vi "Read Write Config File.vi"(4 "Operation":enum16{"Read", "Write"}(ring)=enum."Write", 6 "Config File":T1=enum."General", 8 "error in (no error)":errorcluster, 11 "Section-Key-Value In":string[][](array[string])) -> (0 "error out":errorcluster, 2 "Section-Key-Value Out":string[][](array[string]))   [LabVIEW 2020]
uses:
  Control/Config File Selection.ctl
  <vilib>/Utility/config.llb/Read Key (String).vi
  <vilib>/Utility/config.llb/Write Key (String).vi
  <vilib>/Utility/config.llb/NI_LVConfig.lvlib
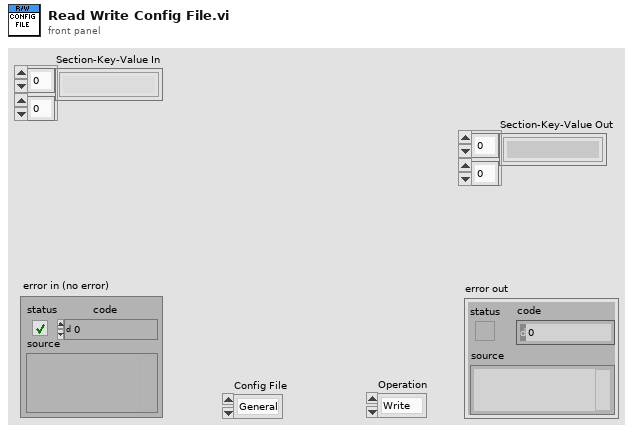
[diagram p1: front panel]
types:
  T1 = typedef "Config File Selection.ctl" = enum16{"Modbus", "SQL", "General"}
  T2 = enum32{"invalid app kind", "Development System", "Run Time System", "Student Edition", "Embedded LabVIEW", "Evaluation", "Custom"}
  T3 = typedef "NI_LVConfig.lvlib/Config Data RefNum.ctl" = refnum<k1>
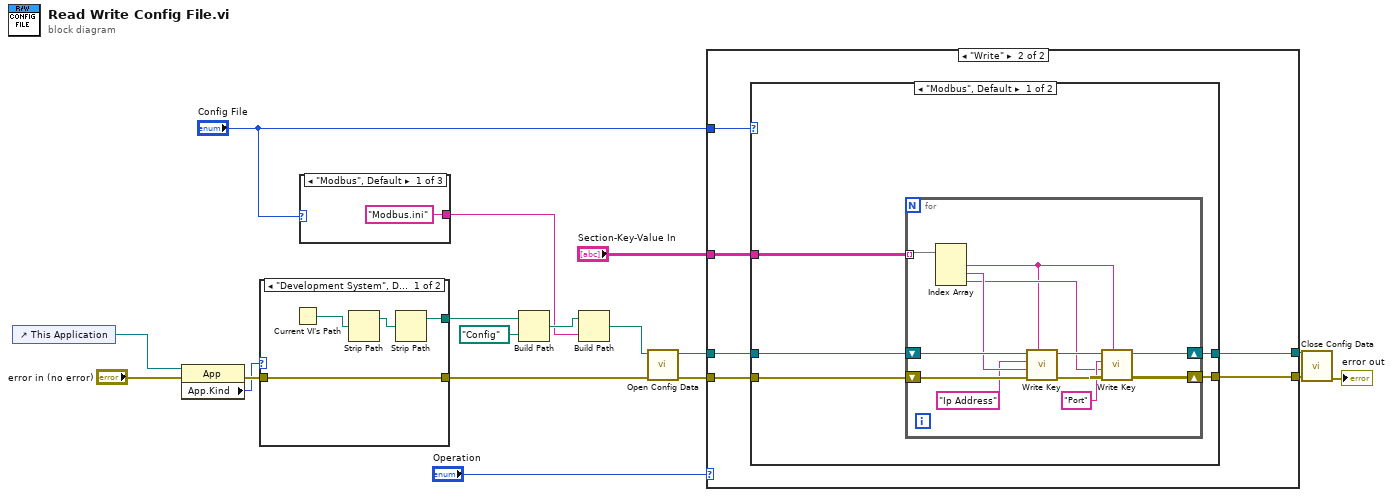
[diagram p0: block diagram]
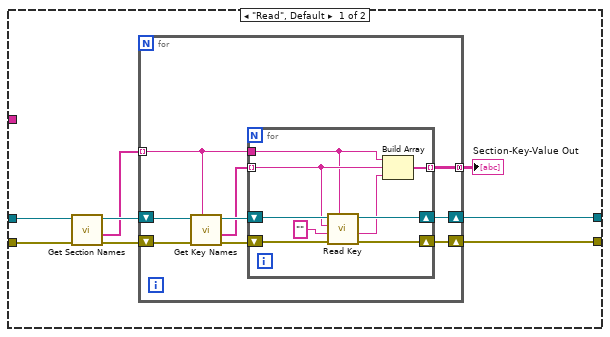
[diagram p2: hidden frame]
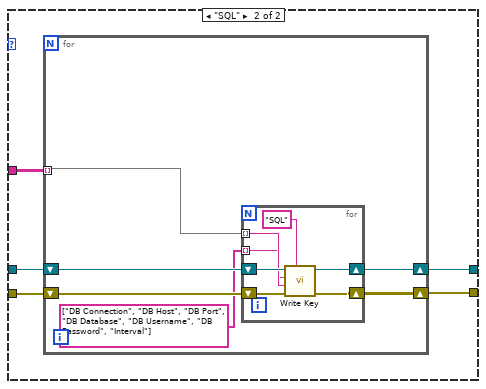
[diagram p3: hidden frame]
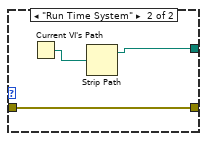
[diagram p4: hidden frame]
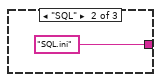
[diagram p5: hidden frame]
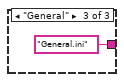
[diagram p6: hidden frame]
diagram:
  n1 = control-ref of="This Application"() -> (w17:refnum<vi>)
  n2 = property class="App"(reference=w17, error in="error in (no error)") -> (error out=w16:errorcluster, "App.Kind"=w15:T2)  [unwired: 1 out]
  n3 = case shown="\"Development System\", Default" w15 {
    tunnel: w16 -> [w19 w23]
    tunnel: [w20 w24] -> w14
    tunnel: [w19 w23] -> w10
    frame "Development System", Default {
      n4 = Current VI's Path() -> (path=w22:path)
      n5 = Strip Path(path=w22) -> (stripped path=w21:path)  [unwired: 1 out]
      n6 = Strip Path(path=w21) -> (stripped path=w20:path)  [unwired: 1 out]
    }
    frame "Run Time System" {
      n7 = Current VI's Path() -> (path=w25:path)
      n8 = Strip Path(path=w25) -> (stripped path=w24:path)  [unwired: 1 out]
    }
  }
  n9 = case shown="\"Modbus\", Default" "Config File" {
    tunnel: ["Modbus.ini" "SQL.ini" "General.ini"] -> w11
    frame "Modbus", Default {
    }
    frame "SQL" {
    }
    frame "General" {
    }
  }
  n10 = Build Path(base path=w14, name or relative path=path "Config") -> (appended path=w12:path)
  n11 = Build Path(base path=w12, name or relative path=w11) -> (appended path=w9:path)
  n12 = call <vilib>:"Open Config Data.vi"("error in (no error)"=w10, "configuration file path"=w9) -> ("error out"=w7:errorcluster, "refnum"=w6:T3)  [unwired: 7 in, 1 out]
  n13 = case shown="\"Write\"" "Operation" {
    tunnel: w7 -> [w35 w59]
    tunnel: w6 -> [w36 w60]
    tunnel: [w30 w57] -> w5
    tunnel: [w29 w58] -> w4
    tunnel: "Config File" -> [_ w56]
    tunnel: "Section-Key-Value In" -> [_ w55]
    frame "Read", Default {
      n14 = call <vilib>:"Get Section Names.vi"("error in (no error)"=w35, "refnum"=w36) -> ("error out"=w34:errorcluster, "section names"=w32:string[], "refnum out"=w33:T3)  [unwired: 7 in]
      n15 = for {
        tunnel: w32 -> [w40] mode=indexing
        shift-right: [w39] -> w29
        shift-left: w33 -> [w45]
        shift-right: [w38] -> w30
        shift-left: w34 -> [w44]
        tunnel: [w37] -> w31 mode=concatenating
        n16 = call <vilib>:"Get Key Names.vi"("section"=w40, "error in (no error)"=w44, "refnum"=w45) -> ("error out"=w43:errorcluster, "key names"=w41:string[], "refnum out"=w42:T3)  [unwired: 5 in, 1 out]
        n17 = for {
          tunnel: w41 -> [w48] mode=indexing
          tunnel: w40 -> [w47]
          shift-right: [w51] -> w39
          shift-left: w42 -> [w54]
          shift-right: [w50] -> w38
          shift-left: w43 -> [w53]
          tunnel: [w46] -> w37 mode=indexing
          n18 = call-poly <vilib>:"Read Key.vi"("section"=w47, "error in (no error)"=w53, "default value"="", "key"=w48, "refnum"=w54) -> ("error out"=w50:errorcluster, "value"=w49:string, "refnum out"=w51:T3)  [unwired: 3 in, 1 out]
          n19 = Build Array(w47, w48, w49) -> (w46:string[])
        }
      }
      "Section-Key-Value Out" <- w31
    }
    frame "Write" {
      n20 = case shown="\"Modbus\", Default" w56 {
        tunnel: w60 -> [w65 w82]
        tunnel: w59 -> [w64 w81]
        tunnel: [w63 w80] -> w58
        tunnel: [w62 w79] -> w57
        tunnel: w55 -> [w61 w78]
        frame "Modbus", Default {
          n21 = for {
            tunnel: w61 -> [w75] mode=indexing
            shift-right: [w70] -> w63
            shift-left: w65 -> [w76]
            shift-right: [w71] -> w62
            shift-left: w64 -> [w77]
            n22 = Index Array(array=w75) -> (element #1=w66:string, element #2=w74:string, element #3=w67:string)  [unwired: 3 in]
            n23 = call-poly <vilib>:"Write Key.vi"("section"=w66, "error in (no error)"=w77, "value"=w74, "key"="Ip Address", "refnum"=w76) -> ("error out"=w72:errorcluster, "refnum out"=w69:T3)  [unwired: 4 in, 1 out]
            n24 = call-poly <vilib>:"Write Key.vi"("section"=w66, "error in (no error)"=w72, "value"=w67, "key"="Port", "refnum"=w69) -> ("error out"=w71:errorcluster, "refnum out"=w70:T3)  [unwired: 4 in, 1 out]
          }
        }
        frame "SQL" {
          n25 = for {
            tunnel: w78 -> [w83] mode=indexing
            shift-right: [w86] -> w80
            shift-left: w82 -> [w87]
            shift-right: [w85] -> w79
            shift-left: w81 -> [w88]
            n26 = for {
              shift-right: [w92] -> w85
              shift-left: w88 -> [w95]
              shift-right: [w93] -> w86
              shift-left: w87 -> [w94]
              tunnel: w83 -> [w91] mode=indexing
              tunnel: string[] ["DB Connection", "DB Host", "DB Port", "DB Database", "DB Username", "DB Password", "Interval"] -> [w90] mode=indexing
              n27 = call-poly <vilib>:"Write Key.vi"("section"="SQL", "error in (no error)"=w95, "value"=w91, "key"=w90, "refnum"=w94) -> ("error out"=w92:errorcluster, "refnum out"=w93:T3)  [unwired: 4 in, 1 out]
            }
          }
        }
      }
    }
  }
  n28 = call <vilib>:"Close Config Data.vi"("error in (no error)"=w5, "refnum"=w4) -> ("error out"=→"error out":errorcluster)  [unwired: 8 in, 1 out]
